vi "Dashboard Main.vi"() -> ()   [LabVIEW 2012]
uses:
  <vilib>/event_ctls.llb/eventvkey.ctl
  <vilib>/Utility/config.llb/Read Key (String).vi
  <vilib>/Utility/config.llb/Read Key (I32).vi
  <vilib>/Utility/config.llb/Write Key (String).vi
  <vilib>/Utility/config.llb/Write Key (I32).vi
  <vilib>/Utility/config.llb/NI_LVConfig.lvlib
panel:
  out "Mode":T1(ring)=enum."Auto Disabled"
  in  "Viewer":enum32{"Camera Image", "Variables"}(tab)
  out "Mbps":dbl format="%#.1g"
  in  "Enable":bool
  in  "DB Camera Config":bool
  out "Mbps":bool
  out "fps":dbl format="%#.1g"
  out "Image Error Message":string="Timeout in Camera Communications"
  out "Camera Image":T2(plugin-control)
  out "Camera Image 2":T2(plugin-control)
  in  "Camera Settings":T3={"Frame Rate"=15, "Compression"=30, "Size"=1} {"Frame Rate" scale=1.0..30.0; "Size" items=["640x480", "320x240", "160x120"]}
  out "Camera IP 2":string
  out "Camera IP":string
  out "fps 2":dbl format="%#.1g"
  out "Mbps 2":dbl format="%#.1g"
  in  "Enable 2":bool
  in  "FR":i32=15
  out "Tree":string(tree)
  in  "Dashboard Tab":enum32{"Operation", "Test", "Checklist"}(tab)
  in  "Slider":dbl(slide) scale=0.0..100.0 scale format="%#_3g"
  in  "On/Off":bool caption="Solenoid"
  in  "Test Name":u16(ring) items=["Select the test to run...", "Example Test", "-------------------------------", "List of tests is built in robot code.", "Replace with your own automated tests."]
  in  "Test Tree":string(tree)
  in  "Motor":cluster{"Value":dbl, "Enable":bool} {"Value" scale=-1.0..1.0 scale format="%#_3g"}
  out "Progress":T4 {"Test Progress" scale=0.0..100.0}
  in  "Rev/Fwd":cluster{"Forward":bool, "Reverse":bool}
  in  "Ring":u16(ring) items=["Auto", "Fixed indoor", "Fixed outdoor 1", "Fixed outdoor 2", "Fixed fluorescent 1", "Fixed fluorescent 2", "Hold current"]
  in  "Listbox":i32(listbox)
  out "Players":i8
  out "Skeleton Picture":picture
  out "Version":string
  out "Buttons 2":cluster{"1":bool, "2":bool, "3":bool}
  out "Kinect 2":cluster{"X":dbl, "Y":dbl, "Z":dbl} {"X" scale=1.0..-1.0; "Y" scale=1.0..-1.0; "Z" scale=1.0..-1.0}
  out "Buttons 1":cluster{"1":bool, "2":bool, "3":bool}
  out "Kinect 1":cluster{"X":dbl, "Y":dbl, "Z":dbl} {"X" scale=1.0..-1.0; "Y" scale=1.0..-1.0; "Z" scale=1.0..-1.0}
  out "Robot IP":string
  out "Battery Value":dbl(slide) scale=0.0..14.0 scale format="%#_2e"
  out "Battery":sgl(graph)
  # "Customize by placing controls and indicators here and name to match\nDashboard Variables on robot."
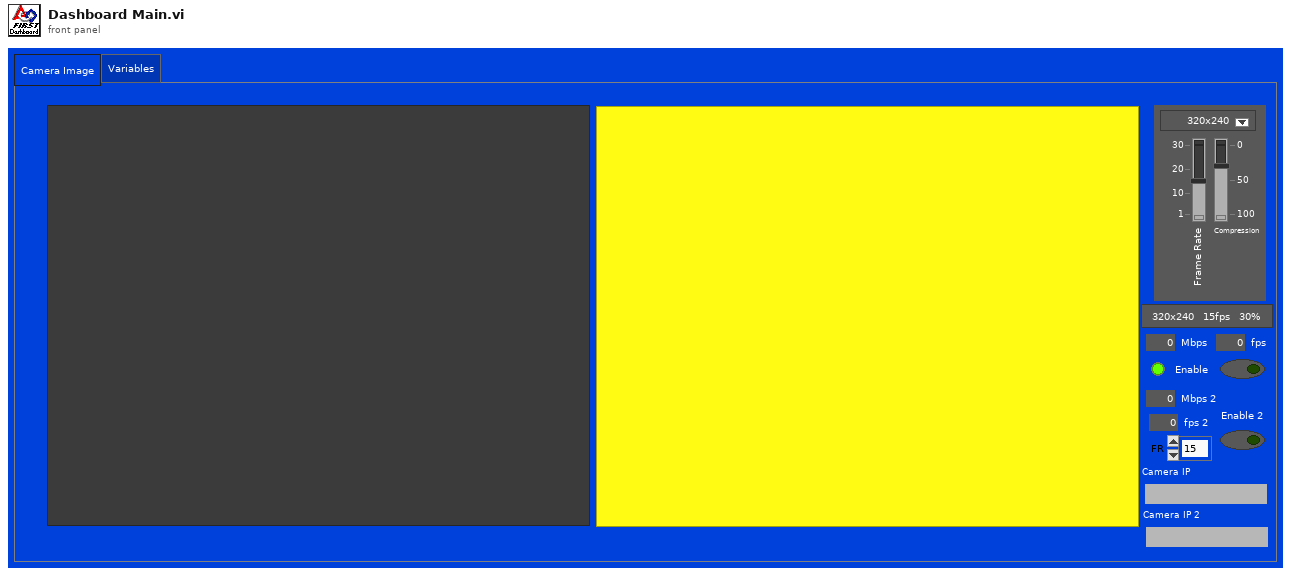
[diagram p1: front panel]
types:
  T1 = enum8{"Tele-Op Disabled", "Tele-Op Enabled", "Auto Disabled", "Auto Enabled", "Test Disabled", "Test Enabled", ""}
  T2 = typedef "IMAQ Image.ctl" = refnum<image>
  T3 = cluster{"Frame Rate":i32, "Compression":i32, "Size":u16}
  T4 = cluster{"Test Progress":u8, "Test Progress Text":string}
  T5 = typedef "Image Type" = u32
  T6 = typedef "LVBoundsTypeDef.ctl" = cluster{"Width":u32, "Height":u32}
  T7 = typedef "SkeletonTrackState.ctl" = enum32{"NotTracked", "PositionOnly", "Tracked"}
  T8 = cluster{"TrackingState":u8[], "Position":cluster{"x":sgl, "y":sgl, "z":sgl}, cluster{"x":sgl, "y":sgl, "z":sgl, sgl}[], "TrackState":T7}
  T9 = cluster{cluster{"ScaledToPercentRange":dbl, "ScaledToPercentRange":dbl, "ScaledToPercentRange":dbl}, cluster{bool, bool, bool}}[]
  T10 = cluster{cluster{"ScaledToPercentRange":dbl, "ScaledToPercentRange":dbl, "ScaledToPercentRange":dbl}, cluster{bool, bool, bool}}
  T11 = cluster{"ScaledToPercentRange":dbl, "ScaledToPercentRange":dbl, "ScaledToPercentRange":dbl}
  T12 = typedef "LVRectTypeDef.ctl" = cluster{"Left":i16, "Top":i16, "Right":i16, "Bottom":i16}
  T13 = cluster{"Competition mode":bool, "Robot Link":bool, "Autonomous":bool, "Enabled":bool, "E-Stop":bool, "Simulated":bool, "TestMode":bool, "Docked Window":bool}
  T14 = typedef "NI_LVConfig.lvlib/Config Data RefNum.ctl" = refnum<k1>
  T15 = typedef "eventvkey.ctl" = enum16{"ASCII", "Enter", "Return", "Shift", "Ctrl", "Alt", "Cmd", "Opt", "Caps", "NumLock", "Clear", "Break", "Up", "Down", "Left", "Right", "Insert", "Delete", "Home", "End", "PageUp", "PageDown", "Escape", "Help", "Pause", "ScrollLock", "F1", "F2", "F3", "F4", "F5", "F6", "F7", "F8", "F9", "F10", "F11", "F12", "F13", "F14", "F15", "F16", "F17", "F18", "F19", "F20", "F21", "F22", "F23", "F24", "Play", "VolumeUp", "VolumeDown", "Mute", "Two Byte Char"}
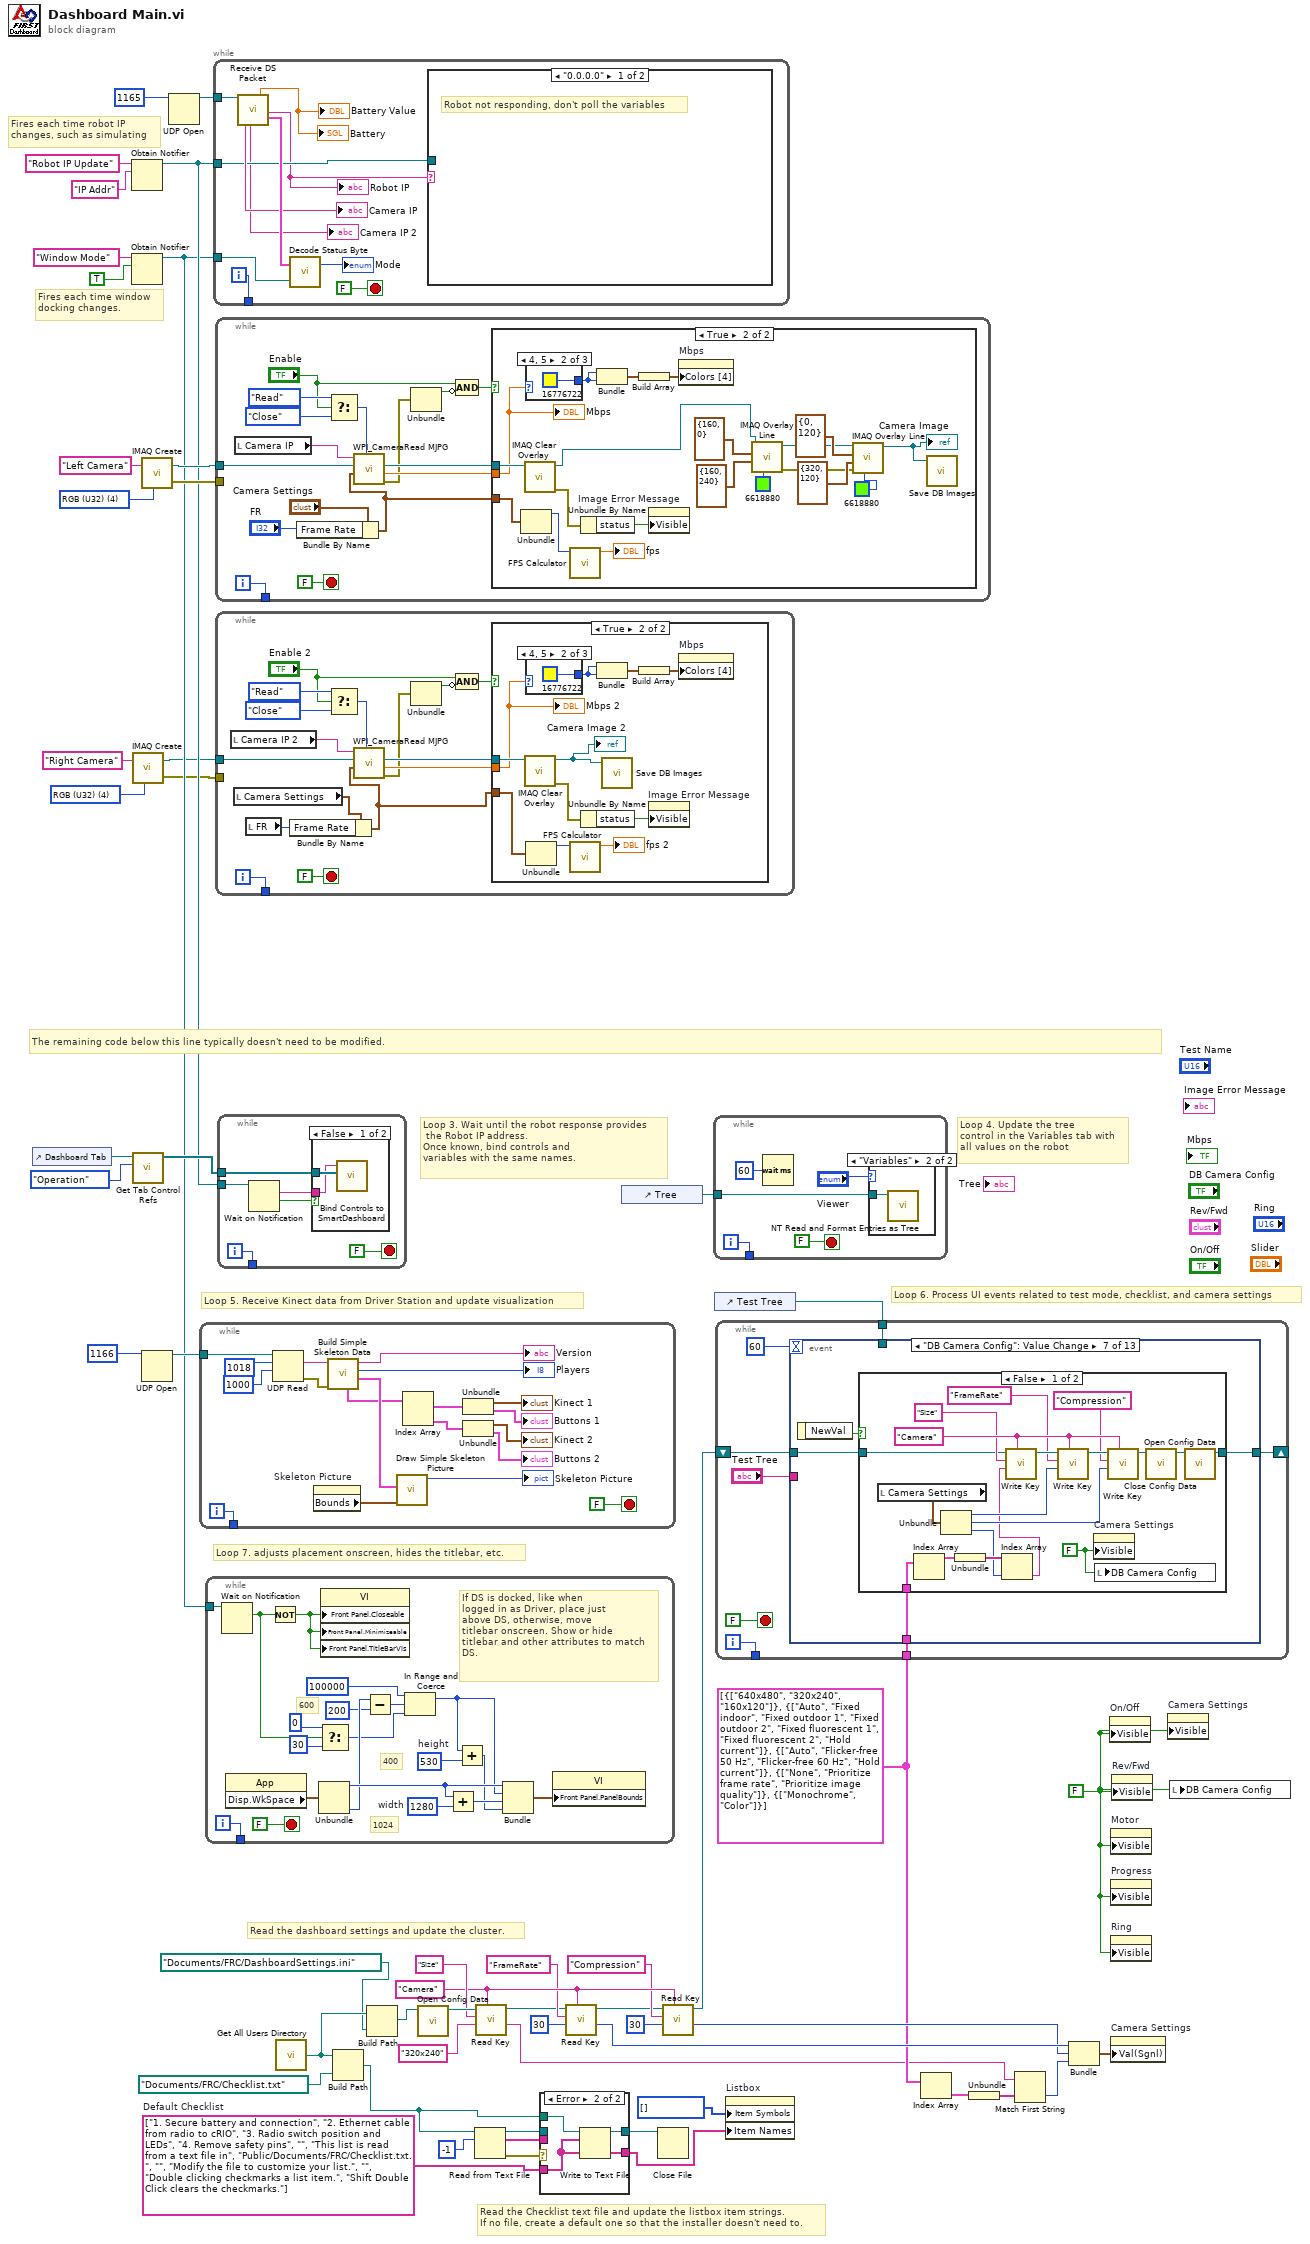
[diagram p0: block diagram]
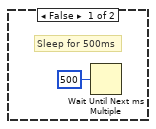
[diagram p2: hidden frame]
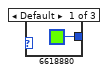
[diagram p3: hidden frame]
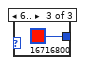
[diagram p4: hidden frame]
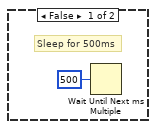
[diagram p6: hidden frame]
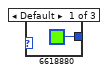
[diagram p7: hidden frame]
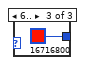
[diagram p8: hidden frame]
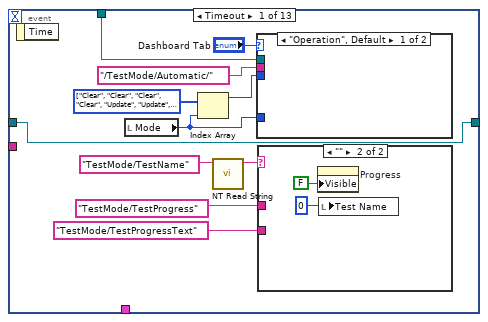
[diagram p10: hidden frame]
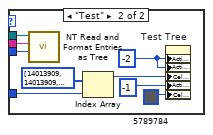
[diagram p11: hidden frame]
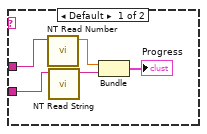
[diagram p12: hidden frame]
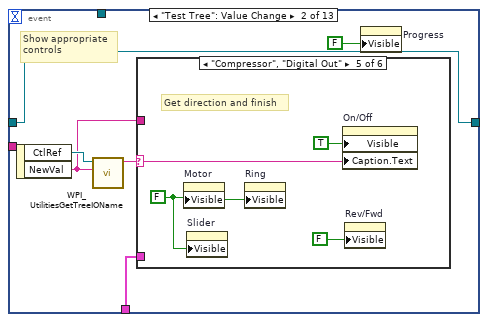
[diagram p13: hidden frame]
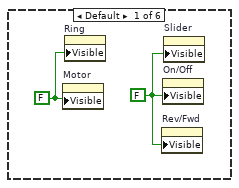
[diagram p14: hidden frame]
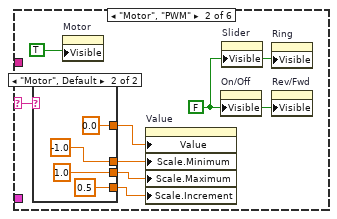
[diagram p15: hidden frame]
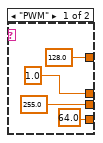
[diagram p16: hidden frame]
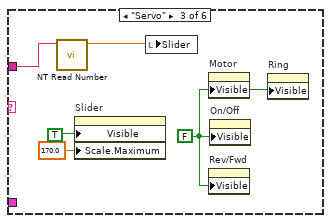
[diagram p17: hidden frame]
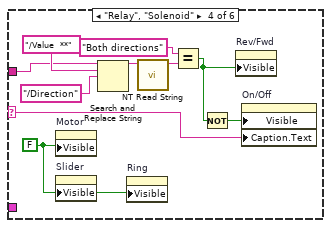
[diagram p18: hidden frame]
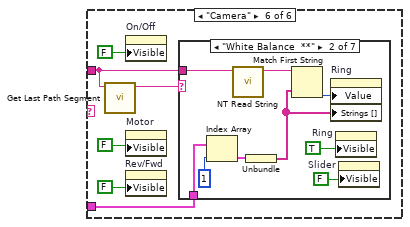
[diagram p19: hidden frame]
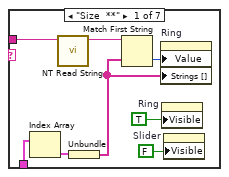
[diagram p20: hidden frame]
diagram:
  w3 = T5 4 items=["Grayscale (U8)", "Grayscale (I16)", "Grayscale (SGL)", "Complex (CSG)", "RGB (U32)", "HSL (U32)", "RGB (U64)"] ("Image Type")
  w25 = "Camera"
  w17 = cluster{string[]}[] [{["640x480", "320x240", "160x120"]}, {["Auto", "Fixed indoor", "Fixed outdoor 1", "Fixed outdoor 2", "Fixed fluorescent 1", "Fixed fluorescent 2", "Hold current"]}, {["Auto", "Flicker-free 50 Hz", "Flicker-free 60 Hz", "Hold current"]}, {["None", "Prioritize frame rate", "Prioritize image quality"]}, {["Monochrome", "Color"]}]
  w33 = string[] ["1. Secure battery and connection", "2. Ethernet cable from radio to cRIO", "3. Radio switch position and LEDs", "4. Remove safety pins", "", "This list is read from a text file in", "Public/Documents/FRC/Checklist.txt.", "", "Modify the file to customize your list.", "", "Double clicking checkmarks a list item.", "Shift Double Click clears the checkmarks."]  # Default Checklist
  w31 = FALSE ("Visible")
  w54 = T5 4 items=["Grayscale (U8)", "Grayscale (I16)", "Grayscale (SGL)", "Complex (CSG)", "RGB (U32)", "HSL (U32)", "RGB (U64)"] ("Image Type")
  # "Fires each time robot IP\nchanges, such as simulating"
  # "Fires each time window\ndocking changes."
  # "Read the Checklist text file and update the listbox item strings.\nIf no file, create a default one so that the installer doesn't need to."
  # "The remaining code below this line typically doesn't need to be modified."
  # "Loop 6. Process UI events related to test mode, checklist, and camera settings"
  # "Read the dashboard settings and update the cluster."
  # "Loop 4. Update the tree\ncontrol in the Variables tab with\nall values on the robot"
  # "Loop 3. Wait until the robot response provides\n the Robot IP address.\nOnce known, bind controls and\nvariables with the same names."
  # "Loop 5. Receive Kinect data from Driver Station and update visualization"
  # "Loop 7. adjusts placement onscreen, hides the titlebar, etc."
  n1 = control-ref of="Dashboard Tab"() -> (w47:refnum<vi>)
  n2 = Obtain Notifier(name (unnamed)="Robot IP Update", notification data type="IP Addr" ("name (unnamed)")) -> (notifier out=w44:refnum<notifier>)  [unwired: 2 in, 2 out]
  n3 = Obtain Notifier(name (unnamed)="Window Mode", notification data type=TRUE) -> (notifier out=w37:refnum<notifier>)  [unwired: 2 in, 2 out]
  n4 = call "IMAQ Create"("Image Name"="Right Camera", "Image Type"=w3) -> ("New Image"=w2:T2, "error out"=w1:errorcluster)  [unwired: 2 in, 1 out]
  n5 = call <vilib>:"Get Tab Control Refs.vi"("Page Index"=enum32{"Operation", "Test"}."Operation" ("Dashboard Tab"), "TabControl in"=w47) -> ("ControlsOnPage"=w48:refnum<vi>[])  [unwired: 9 in]
  n6 = call "IMAQ Create"("Image Name"="Left Camera", "Image Type"=w54) -> ("New Image"=w52:T2, "error out"=w51:errorcluster)  [unwired: 2 in, 1 out]
  n7 = UDP Open(11:u16 1166 ("port")) -> (port=w49:refnum<k16>)  [unwired: 2 in, 4 out]
  n8 = UDP Open(11:u16 1165 ("port")) -> (port=w55:refnum<k16>)  [unwired: 2 in, 4 out]
  n9 = while {
    tunnel: w49 -> [w73]
    tunnel: [w58] -> _
    i -> [w58]
    stop <- FALSE stop-if-true
    n10 = UDP Read(connection ID=w73, max size (548)=1018 ("bytes to read"), timeout ms (25000)=1000) -> (data out=w67:string, error out=w57:errorcluster)  [unwired: 1 in, 3 out]
    n11 = property on="Skeleton Picture" class="Pict"() -> ("Bounds"=w69:T6)  [unwired: 2 in, 2 out]
    n12 = call "Build Simple Skeleton Data.vi"("error in (no error)"=w57, "data in"=w67) -> ("Skeleton Data"=w68:T8, "NumPlayers"=→"Players":i8, "Version String"=→"Version":string, "Simple Joystick Info"=w65:T9)  [unwired: 5 in, 1 out]
    n13 = call "Draw Simple Skeleton Picture.vi"("Bounds"=w69, "Simple Skeleton"=w68) -> ("new picture out"=→"Skeleton Picture":picture)  [unwired: 9 in]
    n14 = Index Array(array=w65) -> (element #1=w64:T10, element #2=w63:T10)  [unwired: 2 in]
    n15 = Unbundle(w64) -> (→"Kinect 1":T11, →"Buttons 1":cluster{bool, bool, bool})
    n16 = Unbundle(w63) -> (→"Kinect 2":T11, →"Buttons 2":cluster{bool, bool, bool})
  }
  n17 = while {
    tunnel: w37 -> [w94]
    tunnel: [w92] -> _
    i -> [w92]
    stop <- FALSE stop-if-true
    w84 = 1280  # width
    w87 = 530  # height
    # "600"
    # "1024"
    # "400"
    # "If DS is docked, like when\nlogged in as Driver, place just\nabove DS, otherwise, move\ntitlebar onscreen. Show or hide\ntitlebar and other attributes to match\nDS."
    n18 = Wait on Notification(notifier=w94) -> (notification=w79:bool)  [unwired: 3 in, 3 out]
    n19 = property class="App"() -> ("Disp.WkSpace"=w90:T12)  [unwired: 2 in, 2 out]
    n20 = Not(x=w79) -> (.not. x?=w93:bool)
    n21 = Unbundle(w90) -> ("Left"=w88:i16, "Bottom"=w85:i16)  [unwired: 2 out]
    n22 = Select(t=0, s=w79, f=30) -> (s? t:f=w78:i32)
    n23 = property class="VI"("Front Panel.Closeable"=w93, "Front Panel.Minimizeable"=w93, "Front Panel.TitleBarVis"=w93) -> ()  [unwired: 2 in, 2 out]
    n24 = Subtract(x=w85, y=200) -> (x-y=w82:i32)
    n25 = In Range and Coerce(upper limit=100000, x=w82, lower limit=w78) -> (coerced(x)=w76:i32)  [unwired: 1 out]
    n26 = Add(x=w88, y=w84) -> (x+y=w89:i32)
    n27 = Add(x=w76, y=w87) -> (x+y=w86:i32)
    n28 = Bundle("Left"=w88, w76, w89, w86) -> (w91:cluster{"Left":i16, i32, i32, i32})  [unwired: 1 out]
    n29 = property class="VI"("Front Panel.PanelBounds"=w91) -> ()  [unwired: 2 in, 2 out]
  }
  n30 = while {
    tunnel: w55 -> [w104]
    tunnel: w44 -> [w98]
    tunnel: w37 -> [w102]
    tunnel: [w99] -> _
    i -> [w99]
    stop <- FALSE stop-if-true
    n31 = call "Receive DS Packet.vi"("Recv Socket"=w104) -> ("Camera IP Address"=→"Camera IP":string, "Camera IP Address 2"=→"Camera IP 2":string, "Battery"=→"Battery" →"Battery Value":sgl, "Robot IP Address"=w97:string, "Status"=w105:T13)  [unwired: 8 in, 6 out]
    "Robot IP" <- w97
    n32 = call "Decode Status Byte.vi"("Window Mode Notifier"=w102, "Status"=w105) -> ("Mode"=→"Mode":T1)  [unwired: 1 out]
    n33 = case shown="\"0.0.0.0\"" w97 {
      selector: w97 -> [_ w107]
      tunnel: w98 -> [_ w108]
      frame "0.0.0.0" {
        # "Robot not responding, don't poll the variables"
      }
      frame Default {
        # "Get info from Code"
        n34 = Send Notification(notification=w107, notifier=w108) -> ()  [unwired: 1 in, 2 out]
      }
    }
  }
  n35 = while {
    tunnel: w52 -> [w121]
    tunnel: w51 -> [_]
    tunnel: [w123] -> _
    i -> [w123]
    stop <- FALSE stop-if-true
    n36 = local read "Camera IP"() -> (w122:string)
    n37 = Bundle By Name(cluster="Camera Settings", "Frame Rate"="FR") -> (w109:T3)
    n38 = Select(t=enum16{"Read", "Reopen", "Close"}."Read" ("Operation"), s="Enable", f=enum16{"Read", "Reopen", "Close"}."Close" ("Operation")) -> (s? t:f=w116:enum16{"Read", "Reopen", "Close"})
    n39 = call <vilib>:"WPI_CameraRead MJPG.vi"("Operation"=w116, "Camera Settings"=w109, "Image"=w121, "address"=w122) -> ("error out"=w115:errorcluster, "Bandwidth (kbps)"=w119:dbl, "Image Out"=w120:T2)  [unwired: 5 in]
    n40 = Unbundle(w115) -> ("status"=w113:bool)  [unwired: 2 out]
    n41 = Compound Arithmetic op=AND("Enable", invert w113) -> (w112:bool)
    n42 = case shown="True" w112 {
      tunnel: w109 -> [_ w137]
      tunnel: w120 -> [_ w140]
      tunnel: w119 -> [_ w139]
      frame False {
        # "Sleep for 500ms"
        n43 = Wait Until Next ms Multiple(millisecond multiple=u32 500) -> ()  [unwired: 1 out]
      }
      frame True {
        n44 = Unbundle(w137) -> ("Frame Rate"=w127:i32)  [unwired: 2 out]
        n45 = call "IMAQ Clear Overlay"("Image"=w140) -> ("error out"=w144:errorcluster, "Image Out"=w129:T2)  [unwired: 2 in, 7 out]
        n46 = case shown="4, 5" w139 {
          tunnel: [u32 6618880 ("Color Box") u32 16776722 ("Color Box") u32 16716800 ("Color Box")] -> w141
          frame Default {
          }
          frame 4, 5 {
          }
          frame 6.. {
          }
        }
        n47 = call "FPS Calculator.vi"("Average Count"=w127) -> ("fps"=→"fps":dbl)  [unwired: 10 in]
        n48 = Unbundle By Name(w144) -> ("status"=w145:bool)
        n49 = Bundle("Color Box"=w141, "Color Box"=w141) -> (w143:cluster{"Color Box":u32, "Color Box":u32})  [unwired: 1 out]
        n50 = Build Array(w143) -> (w142:cluster{"Color Box":u32, "Color Box":u32}[])
        n51 = property on="Image Error Message" class="Str"("Visible"=w145) -> ()  [unwired: 2 in, 2 out]
        n52 = property on="Mbps" class="Bool (strict)"("Colors [4]"=w142) -> ()  [unwired: 2 in, 2 out]
        n53 = call "IMAQ Overlay Line"("Color"=u32 6618880, "End Point"=cluster{"X":i32, "Y":i32} {"X"=160, "Y"=240}, "Start Point"=cluster{"X":i32, "Y":i32} {"X"=160, "Y"=0}, "Image"=w129) -> ("error out"=w134:errorcluster, "Image Out"=w133:T2)  [unwired: 6 in]
        n54 = call "IMAQ Overlay Line"("Color"=u32 6618880, "error in (no error)"=w134, "End Point"=cluster{"X":i32, "Y":i32} {"X"=320, "Y"=120}, "Start Point"=cluster{"X":i32, "Y":i32} {"X"=0, "Y"=120}, "Image"=w133) -> ("Image Out"=w128:T2)  [unwired: 5 in, 1 out]
        "Camera Image" <- w128
        n55 = call "Save DB Images.vi"("Image"=w128) -> ()  [unwired: 2 in, 1 out]
        "Mbps" <- w139
      }
    }
  }
  n56 = while {
    tunnel: w2 -> [w161]
    tunnel: [w163] -> _
    tunnel: w1 -> [_]
    i -> [w163]
    stop <- FALSE stop-if-true
    n57 = local read "Camera IP 2"() -> (w162:string)
    n58 = local read "Camera Settings"() -> (w150:T3)
    n59 = local read "FR"() -> (w151:i32)
    n60 = Bundle By Name(cluster=w150, "Frame Rate"=w151) -> (w149:T3)
    n61 = Select(t=enum16{"Read", "Reopen", "Close"}."Read" ("Operation"), s="Enable 2", f=enum16{"Read", "Reopen", "Close"}."Close" ("Operation")) -> (s? t:f=w156:enum16{"Read", "Reopen", "Close"})
    n62 = call <vilib>:"WPI_CameraRead MJPG.vi"("Operation"=w156, "Camera Settings"=w149, "Image"=w161, "address"=w162) -> ("error out"=w155:errorcluster, "Bandwidth (kbps)"=w159:dbl, "Image Out"=w160:T2)  [unwired: 5 in]
    n63 = Unbundle(w155) -> ("status"=w153:bool)  [unwired: 2 out]
    n64 = Compound Arithmetic op=AND("Enable 2", invert w153) -> (w152:bool)
    n65 = case shown="True" w152 {
      tunnel: w149 -> [_ w168]
      tunnel: w160 -> [_ w171]
      tunnel: w159 -> [_ w170]
      frame False {
        # "Sleep for 500ms"
        n66 = Wait Until Next ms Multiple(millisecond multiple=u32 500) -> ()  [unwired: 1 out]
      }
      frame True {
        n67 = call "IMAQ Clear Overlay"("Image"=w171) -> ("error out"=w175:errorcluster, "Image Out"=w166:T2)  [unwired: 2 in, 7 out]
        "Camera Image 2" <- w166
        n68 = case shown="4, 5" w170 {
          tunnel: [u32 6618880 ("Color Box") u32 16776722 ("Color Box") u32 16716800 ("Color Box")] -> w172
          frame Default {
          }
          frame 4, 5 {
          }
          frame 6.. {
          }
        }
        n69 = Unbundle(w168) -> ("Frame Rate"=w167:i32)  [unwired: 2 out]
        n70 = call "FPS Calculator.vi"("Average Count"=w167) -> ("fps"=→"fps 2":dbl)  [unwired: 10 in]
        n71 = Unbundle By Name(w175) -> ("status"=w176:bool)
        n72 = Bundle("Color Box"=w172, "Color Box"=w172) -> (w174:cluster{"Color Box":u32, "Color Box":u32})  [unwired: 1 out]
        n73 = call "Save DB Images.vi"("Image"=w166) -> ()  [unwired: 2 in, 1 out]
        n74 = Build Array(w174) -> (w173:cluster{"Color Box":u32, "Color Box":u32}[])
        n75 = property on="Image Error Message" class="Str"("Visible"=w176) -> ()  [unwired: 2 in, 2 out]
        n76 = property on="Mbps" class="Bool (strict)"("Colors [4]"=w173) -> ()  [unwired: 2 in, 2 out]
        "Mbps 2" <- w170
      }
    }
  }
  n77 = while {
    tunnel: w48 -> [w185]
    tunnel: w44 -> [w182]
    tunnel: [w180] -> _
    i -> [w180]
    stop <- FALSE stop-if-true
    n78 = Wait on Notification(notifier=w182) -> (notification=w181:string, timed out?=w183:bool)  [unwired: 3 in, 2 out]
    n79 = case shown="False" w183 {
      tunnel: w185 -> [w187 _]
      tunnel: w181 -> [w186 _]
      frame False {
        n80 = call <vilib>:"Bind Controls to SmartDashboard.vi"("Bound Control Refs"=w187, "Server IP Address"=w186) -> ()  [unwired: 10 in]
      }
      frame True {
      }
    }
  }
  n81 = call "Get All Users Directory.vi"() -> ("All User Path"=w30:path)
  n82 = Build Path(base path=w30, name or relative path=path "Documents/FRC/Checklist.txt") -> (appended path=w34:path)
  n83 = Build Path(base path=w30, name or relative path=path "Documents/FRC/DashboardSettings.ini") -> (appended path=w29:path)
  n84 = call <vilib>:"Open Config Data.vi"("configuration file path"=w29) -> ("refnum"=w28:T14)  [unwired: 8 in, 2 out]
  n85 = Read from Text File(file (use dialog)=w34, count=-1 ("timeout ms (25000)")) -> (refnum out=w12:refnum<file>, text=w35:string[], error out=w36:errorcluster)  [unwired: 2 in, 1 out]
  n86 = call-poly <vilib>:"Read Key.vi"("section"=w25, "default value"="320x240", "key"="Size", "refnum"=w28) -> ("value"=w15:string, "refnum out"=w10:T14)  [unwired: 2 in, 4 out]
  n87 = case shown="Error" w36 {
    tunnel: w35 -> [w189 _]
    tunnel: [w189 w191] -> w32
    tunnel: w33 -> [_ w191]
    tunnel: w34 -> [_ w192]
    tunnel: [w188 w190] -> w11
    tunnel: w12 -> [w188 _]
    frame No Error {
    }
    frame Error {
      n88 = Write to Text File(file (use dialog)=w192, text=w191) -> (refnum out=w190:refnum<file>)  [unwired: 2 in, 2 out]
    }
  }
  n89 = call-poly <vilib>:"Read Key.vi"("section"=w25, "default value"=30, "key"="FrameRate", "refnum"=w10) -> ("value"=w20:i32, "refnum out"=w9:T14)  [unwired: 1 in, 5 out]
  n90 = control-ref of="Tree"() -> (w6:refnum<vi>)
  n91 = Close File(refnum=w11) -> ()  [unwired: 1 in, 2 out]
  n92 = call-poly <vilib>:"Read Key.vi"("section"=w25, "default value"=30, "key"="Compression", "refnum"=w9) -> ("value"=w19:i32, "refnum out"=w7:T14)  [unwired: 1 in, 5 out]
  n93 = while {
    tunnel: [w194] -> _
    tunnel: w6 -> [w193]
    i -> [w194]
    stop <- FALSE stop-if-true
    n94 = Wait (ms)(milliseconds to wait=u32 60) -> ()  [unwired: 1 out]
    n95 = case shown="\"Variables\"" "Viewer" {
      tunnel: w193 -> [_ w198]
      frame Default {
      }
      frame "Variables" {
        n96 = call <vilib>:"NT Read and Format Entries as Tree.vi"("Tree Refnum"=w198) -> ()  [unwired: 9 in, 2 out]
      }
    }
  }
  n97 = control-ref of="Test Tree"() -> (w5:refnum<vi>)
  n98 = while {
    tunnel: w17 -> [w203]
    shift-right: [w202] -> _
    shift-left: w7 -> [w201]
    tunnel: [w200] -> _
    tunnel: w5 -> [w199]
    i -> [w200]
    stop <- FALSE stop-if-true
    n99 = event shown="[6] \"DB Camera Config\": Value Change" {
      selector: _ -> [_ _ _ _ _ _ _ _ _ _ _ _ _]
      dyn-events: _ -> [_ _ _ _ _ _ _ _ _ _ _ _ _]
      timeout: u32 60 ("milliseconds to wait") -> [_ _ _ _ _ _ _ _ _ _ _ _ _]
      tunnel: w199 -> [w213 _ _ _ _ _ _ _ _ _ _ _ _]
      tunnel: "Test Tree" -> [_ _ _ _ _ _ _ _ w407 w415 w417 w421 w429]
      tunnel: w203 -> [_ w235 _ _ _ _ w371 w401 _ _ _ _ _]
      tunnel: [w207 w234 _ w337 w345 w357 w370 w394 w406 w413 w416 w420 w428] -> w202
      tunnel: w201 -> [w207 w234 _ w337 w345 w357 w369 w394 w406 w413 w416 w420 w428]
      event Timeout {
        w212 = enum16{"Update", "Clear"}[] [enum."Clear", enum."Clear", enum."Clear", enum."Clear", enum."Update", enum."Update", enum."Clear"] items=["Update", "Clear"]
        n100 = event-data() -> ()  [unwired: 1 in, 1 out]
        n101 = local read "Mode"() -> (w210:T1)
        n102 = Index Array(array=w212, index=w210) -> (element=w211:enum16{"Update", "Clear"})
        n103 = call <vilib>:"NT Read String.vi"("Name"="TestMode/TestName") -> ("String"=w216:string)  [unwired: 9 in, 1 out]
        n104 = case shown="\"Operation\", Default" "Dashboard Tab" {
          tunnel: w213 -> [_ w226]
          tunnel: "/TestMode/Automatic/" ("Name Pattern") -> [_ w225]
          tunnel: w211 -> [_ w224]
          tunnel: w210 -> [_ w222]
          frame "Operation", Default {
          }
          frame "Test" {
            w221 = -2 ("Active Item:Row Number")
            n105 = call <vilib>:"NT Read and Format Entries as Tree.vi"("Operation"=w224, "Name Pattern"=w225, "Tree Refnum"=w226) -> ()  [unwired: 7 in, 2 out]
            n106 = Index Array(array=u32[] [14013909, 14013909, 14013909, 14013909, 14013909, 16777215, 14013909], index=w222) -> (element=w220:u32)
            n107 = property on="Test Tree" class="Tree (strict)"("Active Item Row Number"=w221, "ActiveColNum"=w221, "CellBG"=w220, "Active Item Row Number"=-1 ("Active Item:Row Number"), "CellBG"=u32 5789784 ("Color Box")) -> ()  [unwired: 2 in, 2 out]
          }
        }
        n108 = case shown="\"\"" w216 {
          tunnel: "TestMode/TestProgress" ("Name") -> [w228 _]
          tunnel: "TestMode/TestProgressText" ("Name") -> [w227 _]
          frame Default {
            n109 = call <vilib>:"NT Read Number.vi"("Name"=w228) -> ("Numeric"=w229:dbl)  [unwired: 9 in, 1 out]
            n110 = call <vilib>:"NT Read String.vi"("Name"=w227) -> ("String"=w230:string)  [unwired: 9 in, 1 out]
            n111 = Bundle("Numeric"=w229, "String"=w230) -> (→"Progress":cluster{"Numeric":dbl, "String":string})  [unwired: 1 in]
          }
          frame "" {
            n112 = property on="Progress" class="Clust (strict)"("Visible"=FALSE) -> ()  [unwired: 2 in, 2 out]
            n113 = local write "Test Name"(u16 0) -> ()
          }
        }
      }
      event "Test Tree": Value Change {
        # "Show appropriate\ncontrols"
        n114 = event-data() -> ("CtlRef"=w238:refnum<vi>, "NewVal"=w236:string)  [unwired: 1 in]
        n115 = call <vilib>:"WPI_UtilitiesGetTreeIOName.vi"("NewVal"=w236, "TreeControl in"=w238) -> ("I/O Name"=w239:string)  [unwired: 9 in]
        n116 = case shown="\"Compressor\", \"Digital Out\"" w239 {
          selector: w239 -> [_ w246 _ w264 w273 _]
          tunnel: w236 -> [_ _ w261 w263 _ w280]
          tunnel: w235 -> [_ _ _ _ _ w279]
          frame Default {
            w241 = FALSE ("Visible")
            w240 = FALSE ("Visible")
            n117 = property on="Motor" class="Clust (strict)"("Visible"=w240) -> ()  [unwired: 2 in, 2 out]
            n118 = property on="Ring" class="Ring (strict)"("Visible"=w240) -> ()  [unwired: 2 in, 2 out]
            n119 = property on="Rev/Fwd" class="Clust (strict)"("Visible"=w241) -> ()  [unwired: 2 in, 2 out]
            n120 = property on="On/Off" class="Bool (strict)"("Visible"=w241) -> ()  [unwired: 2 in, 2 out]
            n121 = property on="Slider" class="Slide (strict)"("Visible"=w241) -> ()  [unwired: 2 in, 2 out]
          }
          frame "Motor", "PWM" {
            w247 = FALSE ("Visible")
            n122 = case shown="\"Motor\", Default" w246 {
              tunnel: [1.0 ("Value") -1.0 ("Value")] -> w245
              tunnel: [255.0 ("Value") 1.0 ("Value")] -> w244
              tunnel: [128.0 ("Value") 0.0 ("Value")] -> w243
              tunnel: [64.0 ("Value") 0.5 ("Value")] -> w242
              frame "PWM" {
              }
              frame "Motor", Default {
              }
            }
            n123 = property on="Motor" class="Clust (strict)"("Visible"=TRUE) -> ()  [unwired: 2 in, 2 out]
            n124 = property on="Value" class="Slide (strict)"("Value"=w243, "Scale.Minimum"=w245, "Scale.Maximum"=w244, "Scale.Increment"=w242) -> ()  [unwired: 2 in, 2 out]
            n125 = property on="On/Off" class="Bool (strict)"("Visible"=w247) -> ()  [unwired: 2 in, 2 out]
            n126 = property on="Slider" class="Slide (strict)"("Visible"=w247) -> ()  [unwired: 2 in, 2 out]
            n127 = property on="Ring" class="Ring (strict)"("Visible"=w247) -> ()  [unwired: 2 in, 2 out]
            n128 = property on="Rev/Fwd" class="Clust (strict)"("Visible"=w247) -> ()  [unwired: 2 in, 2 out]
          }
          frame "Servo" {
            w259 = FALSE ("Visible")
            n129 = call <vilib>:"NT Read Number.vi"("Name"=w261) -> ("Numeric"=w260:dbl)  [unwired: 9 in, 1 out]
            n130 = property on="Slider" class="Slide (strict)"("Visible"=TRUE, "Scale.Maximum"=170.0 ("Scale.Range:Maximum")) -> ()  [unwired: 2 in, 2 out]
            n131 = local write "Slider"(w260) -> ()
            n132 = property on="Motor" class="Clust (strict)"("Visible"=w259) -> ()  [unwired: 2 in, 2 out]
            n133 = property on="Rev/Fwd" class="Clust (strict)"("Visible"=w259) -> ()  [unwired: 2 in, 2 out]
            n134 = property on="On/Off" class="Bool (strict)"("Visible"=w259) -> ()  [unwired: 2 in, 2 out]
            n135 = property on="Ring" class="Ring (strict)"("Visible"=w259) -> ()  [unwired: 2 in, 2 out]
          }
          frame "Relay", "Solenoid" {
            w262 = FALSE ("Visible")
            n136 = property on="Motor" class="Clust (strict)"("Visible"=w262) -> ()  [unwired: 2 in, 2 out]
            n137 = property on="Slider" class="Slide (strict)"("Visible"=w262) -> ()  [unwired: 2 in, 2 out]
            n138 = Search and Replace String(input string=w263, search string="/Value  **", replace string="/Direction") -> (result string=w269:string)  [unwired: 5 in, 3 out]
            n139 = property on="Ring" class="Ring (strict)"("Visible"=w262) -> ()  [unwired: 2 in, 2 out]
            n140 = call <vilib>:"NT Read String.vi"("Name"=w269) -> ("String"=w267:string)  [unwired: 9 in, 1 out]
            n141 = Equal?(x="Both directions", y=w267) -> (x = y?=w265:bool)
            n142 = Not(x=w265) -> (.not. x?=w266:bool)
            n143 = property on="Rev/Fwd" class="Clust (strict)"("Visible"=w265) -> ()  [unwired: 2 in, 2 out]
            n144 = property on="On/Off" class="Bool (strict)"("Visible"=w266, "Caption.Text"=w264) -> ()  [unwired: 2 in, 2 out]
          }
          frame "Compressor", "Digital Out" {
            w272 = FALSE ("Visible")
            # "Get direction and finish"
            n145 = property on="Motor" class="Clust (strict)"("Visible"=w272) -> ()  [unwired: 2 in, 2 out]
            n146 = property on="Slider" class="Slide (strict)"("Visible"=w272) -> ()  [unwired: 2 in, 2 out]
            n147 = property on="Ring" class="Ring (strict)"("Visible"=w272) -> ()  [unwired: 2 in, 2 out]
            n148 = property on="On/Off" class="Bool (strict)"("Visible"=TRUE, "Caption.Text"=w273) -> ()  [unwired: 2 in, 2 out]
            n149 = property on="Rev/Fwd" class="Clust (strict)"("Visible"=FALSE) -> ()  [unwired: 2 in, 2 out]
          }
          frame "Camera" {
            n150 = call <vilib>:"Get Last Path Segment.vi"("String in"=w280) -> ("String out"=w281:string)  [unwired: 10 in]
            n151 = property on="On/Off" class="Bool (strict)"("Visible"=FALSE) -> ()  [unwired: 2 in, 2 out]
            n152 = property on="Motor" class="Clust (strict)"("Visible"=FALSE) -> ()  [unwired: 2 in, 2 out]
            n153 = property on="Rev/Fwd" class="Clust (strict)"("Visible"=FALSE) -> ()  [unwired: 2 in, 2 out]
            n154 = case shown="\"White Balance  **\"" w281 {
              tunnel: w280 -> [w287 w296 w305 w314 w323 _ w329]
              tunnel: w279 -> [w285 w293 w302 w311 w320 _ _]
              frame "Size  **" {
                n155 = Index Array(array=w285) -> (element=w284:cluster{string[]})  [unwired: 1 in]
                n156 = call <vilib>:"NT Read String.vi"("Name"=w287) -> ("String"=w286:string)  [unwired: 9 in, 1 out]
                n157 = Unbundle(w284) -> (w282:string[])
                n158 = Match First String(2:w282, 3:w286) -> (0:w283:i32)  [unwired: 1 out]
                n159 = property on="Ring" class="Ring (strict)"("Value"=w283, "Strings []"=w282) -> ()  [unwired: 2 in, 2 out]
                n160 = property on="Ring" class="Ring (strict)"("Visible"=TRUE) -> ()  [unwired: 2 in, 2 out]
                n161 = property on="Slider" class="Slide (strict)"("Visible"=FALSE) -> ()  [unwired: 2 in, 2 out]
              }
              frame "White Balance  **" {
                n162 = Index Array(array=w293, index=1) -> (element=w294:cluster{string[]})
                n163 = call <vilib>:"NT Read String.vi"("Name"=w296) -> ("String"=w295:string)  [unwired: 9 in, 1 out]
                n164 = Unbundle(w294) -> (w291:string[])
                n165 = Match First String(2:w291, 3:w295) -> (0:w290:i32)  [unwired: 1 out]
                n166 = property on="Ring" class="Ring (strict)"("Value"=w290, "Strings []"=w291) -> ()  [unwired: 2 in, 2 out]
                n167 = property on="Ring" class="Ring (strict)"("Visible"=TRUE) -> ()  [unwired: 2 in, 2 out]
                n168 = property on="Slider" class="Slide (strict)"("Visible"=FALSE) -> ()  [unwired: 2 in, 2 out]
              }
              frame "Exposure  **" {
                n169 = Index Array(array=w302, index=2) -> (element=w303:cluster{string[]})
                n170 = call <vilib>:"NT Read String.vi"("Name"=w305) -> ("String"=w304:string)  [unwired: 9 in, 1 out]
                n171 = Unbundle(w303) -> (w299:string[])
                n172 = Match First String(2:w299, 3:w304) -> (0:w300:i32)  [unwired: 1 out]
                n173 = property on="Ring" class="Ring (strict)"("Value"=w300, "Strings []"=w299) -> ()  [unwired: 2 in, 2 out]
                n174 = property on="Ring" class="Ring (strict)"("Visible"=TRUE) -> ()  [unwired: 2 in, 2 out]
                n175 = property on="Slider" class="Slide (strict)"("Visible"=FALSE) -> ()  [unwired: 2 in, 2 out]
              }
              frame "Exposure Priority  **" {
                n176 = Index Array(array=w311, index=3) -> (element=w312:cluster{string[]})
                n177 = call <vilib>:"NT Read String.vi"("Name"=w314) -> ("String"=w313:string)  [unwired: 9 in, 1 out]
                n178 = Unbundle(w312) -> (w308:string[])
                n179 = Match First String(2:w308, 3:w313) -> (0:w309:i32)  [unwired: 1 out]
                n180 = property on="Ring" class="Ring (strict)"("Value"=w309, "Strings []"=w308) -> ()  [unwired: 2 in, 2 out]
                n181 = property on="Ring" class="Ring (strict)"("Visible"=TRUE) -> ()  [unwired: 2 in, 2 out]
                n182 = property on="Slider" class="Slide (strict)"("Visible"=FALSE) -> ()  [unwired: 2 in, 2 out]
              }
              frame "Color Enable  **" {
                n183 = Index Array(array=w320, index=4) -> (element=w321:cluster{string[]})
                n184 = call <vilib>:"NT Read String.vi"("Name"=w323) -> ("String"=w322:string)  [unwired: 9 in, 1 out]
                n185 = Unbundle(w321) -> (w317:string[])
                n186 = Match First String(2:w317, 3:w322) -> (0:w318:i32)  [unwired: 1 out]
                n187 = property on="Ring" class="Ring (strict)"("Value"=w318, "Strings []"=w317) -> ()  [unwired: 2 in, 2 out]
                n188 = property on="Ring" class="Ring (strict)"("Visible"=TRUE) -> ()  [unwired: 2 in, 2 out]
                n189 = property on="Slider" class="Slide (strict)"("Visible"=FALSE) -> ()  [unwired: 2 in, 2 out]
              }
              frame Default {
                n190 = property on="Ring" class="Ring (strict)"("Visible"=FALSE) -> ()  [unwired: 2 in, 2 out]
                n191 = property on="Slider" class="Slide (strict)"("Visible"=FALSE) -> ()  [unwired: 2 in, 2 out]
              }
              frame "Brightness  **", "Color Level  **", "Compression  **", "FPS  **", "Sharpness  **" {
                n192 = call <vilib>:"NT Read Number.vi"("Name"=w329) -> ("Numeric"=w328:dbl)  [unwired: 9 in, 1 out]
                n193 = local write "Slider"(w328) -> ()
                n194 = property on="Slider" class="Slide (strict)"("Visible"=TRUE, "Scale.Maximum"=100.0 ("Scale.Range:Maximum")) -> ()  [unwired: 2 in, 2 out]
                n195 = property on="Ring" class="Ring (strict)"("Visible"=FALSE) -> ()  [unwired: 2 in, 2 out]
              }
            }
          }
        }
        n196 = property on="Progress" class="Clust (strict)"("Visible"=FALSE) -> ()  [unwired: 2 in, 2 out]
      }
      event "Test Name": Mouse Enter {
        # "Populate the ring with the list of tests"
        n197 = event-data() -> ()  [unwired: 1 in, 1 out]
        n198 = call <vilib>:"NT Read String Array.vi"("Name"="TestMode/TestList") -> ("String Array"=w336:string[])  [unwired: 9 in, 1 out]
        n199 = Build Array (concatenate)("Select the test to run...", w336) -> (w335:string[])
        n200 = property on="Test Name" class="Ring (strict)"("Strings []"=w335) -> ()  [unwired: 2 in, 2 out]
      }
      event "Test Name": Value Change {
        w338 = FALSE ("Visible")
        # "Tell the robot the test name to run"
        n201 = event-data() -> ("NewVal"=w342:u16)  [unwired: 1 in]
        n202 = property on="Test Name" class="Ring (strict)"() -> ("Strings []"=w343:string[])  [unwired: 2 in, 2 out]
        n203 = local write "Progress"(T4 {"Test Progress"=0, "Test Progress Text"=""} ("Progress")) -> ()
        n204 = Index Array(array=w343, index=w342) -> (element=w341:string)
        n205 = call <vilib>:"NT Write String.vi"("String"=w341, "Name"="TestMode/TestName") -> ()  [unwired: 9 in, 1 out]
        n206 = property on="Progress" class="Clust (strict)"("Visible"=TRUE) -> ()  [unwired: 2 in, 2 out]
        n207 = property on="Motor" class="Clust (strict)"("Visible"=w338) -> ()  [unwired: 2 in, 2 out]
        n208 = property on="Slider" class="Slide (strict)"("Visible"=w338) -> ()  [unwired: 2 in, 2 out]
        n209 = property on="On/Off" class="Bool (strict)"("Visible"=w338) -> ()  [unwired: 2 in, 2 out]
        n210 = property on="Rev/Fwd" class="Clust (strict)"("Visible"=w338) -> ()  [unwired: 2 in, 2 out]
        n211 = property on="Ring" class="Ring (strict)"("Visible"=w338) -> ()  [unwired: 2 in, 2 out]
      }
      event "Listbox": Double Click {
        n212 = event-data() -> ("PlatMods.Shift"=w346:bool, "Row"=w348:i32)  [unwired: 1 in]
        n213 = case shown="False" w346 {
          tunnel: w348 -> [w352 _]
          tunnel: 1 -> [w351 _]
          frame False {
            n214 = property on="Listbox" class="LstBox (strict)"() -> ("Item Symbols"=w350:i32[])  [unwired: 2 in, 2 out]
            n215 = Replace Array Subset(array=w350, new element=w351, index=w352) -> (w349:i32[])
            n216 = property on="Listbox" class="LstBox (strict)"("Item Symbols"=w349) -> ()  [unwired: 2 in, 2 out]
          }
          frame True {
            w353 = 0 ("Top Row")
            n217 = property on="Listbox" class="LstBox (strict)"() -> ("Number of Rows"=w355:u32)  [unwired: 2 in, 2 out]
            n218 = Initialize Array(0, w355) -> (w354:i32[])
            n219 = property on="Listbox" class="LstBox (strict)"("Top Row"=w353, "Value"=w353, "Item Symbols"=w354) -> ()  [unwired: 2 in, 2 out]
          }
        }
      }
      event "Listbox": Key Down {
        n220 = event-data() -> ("VKey"=w359:T15)  [unwired: 1 in]
        n221 = case shown="\"Left\", \"Right\"" w359 {
          selector: w359 -> [w364 _]
          tunnel: eventvkey."Left" ("VKey") -> [w362 _]
          frame "Left", "Right" {
            n222 = Equal?(x=w362, y=w364) -> (x = y?=w363:bool)
            n223 = Select(t=0, s=w363, f=1) -> (s? t:f=w365:i32)
            n224 = property on="Listbox" class="LstBox (strict)"() -> ("Item Symbols"=w368:i32[])  [unwired: 2 in, 2 out]
            n225 = Replace Array Subset(array=w368, new element=w365, index="Listbox") -> (w367:i32[])
            n226 = property on="Listbox" class="LstBox (strict)"("Item Symbols"=w367) -> ()  [unwired: 2 in, 2 out]
          }
          frame Default {
          }
        }
      }
      event "DB Camera Config": Value Change {
        n227 = event-data() -> ("NewVal"=w372:bool)  [unwired: 1 in]
        n228 = case shown="False" w372 {
          tunnel: w371 -> [w381 _]
          tunnel: [w374 w392] -> w370
          tunnel: w369 -> [w373 w392]
          frame False {
            w388 = "Camera"
            w391 = FALSE ("Visible")
            n229 = local read "Camera Settings"() -> (w380:T3)
            n230 = Index Array(array=w381) -> (element=w384:cluster{string[]})  [unwired: 1 in]
            n231 = Unbundle(w380) -> ("Frame Rate"=w379:i32, "Compression"=w378:i32, "Size"=w382:u16)
            n232 = Unbundle(w384) -> (w383:string[])
            n233 = Index Array(array=w383, index=w382) -> (element=w377:string)
            n234 = call-poly <vilib>:"Write Key.vi"("section"=w388, "value"=w377, "key"="Size", "refnum"=w373) -> ("refnum out"=w390:T14)  [unwired: 2 in, 5 out]
            n235 = call-poly <vilib>:"Write Key.vi"("section"=w388, "value"=w379, "key"="FrameRate", "refnum"=w390) -> ("refnum out"=w389:T14)  [unwired: 1 in, 6 out]
            n236 = property on="Camera Settings" class="Clust (strict)"("Visible"=w391) -> ()  [unwired: 2 in, 2 out]
            n237 = local write "DB Camera Config"(w391) -> ()
            n238 = call-poly <vilib>:"Write Key.vi"("section"=w388, "value"=w378, "key"="Compression", "refnum"=w389) -> ("refnum out"=w375:T14)  [unwired: 1 in, 6 out]
            n239 = call <vilib>:"Close Config Data.vi"("refnum"=w375) -> ("file path"=w376:path)  [unwired: 2 in, 8 out]
            n240 = call <vilib>:"Open Config Data.vi"("configuration file path"=w376) -> ("refnum"=w374:T14)  [unwired: 8 in, 2 out]
          }
          frame True {
            n241 = property on="Camera Settings" class="Clust (strict)"("Visible"=TRUE) -> ()  [unwired: 2 in, 2 out]
          }
        }
      }
      event "Camera Settings": Value Change {
        n242 = event-data() -> ("NewVal"=w405:T3)  [unwired: 1 in]
        n243 = Index Array(array=w401) -> (element=w400:cluster{string[]})  [unwired: 1 in]
        n244 = Unbundle(w405) -> ("Frame Rate"=w396:i32, "Compression"=w395:i32, "Size"=w398:u16)
        n245 = Unbundle(w400) -> (w399:string[])
        n246 = Index Array(array=w399, index=w398) -> (element=w397:string)
        n247 = Format Into String(format string="%s   %dfps   %d%%", w397, w396, w395) -> (resulting string=w402:string)  [unwired: 2 in, 1 out]
        n248 = Build Array(w402) -> (w403:string[])
        n249 = property on="DB Camera Config" class="Bool (strict)"("Strings [4]"=w403) -> ()  [unwired: 2 in, 2 out]
      }
      event "Motor.Enable": Value Change {
        n250 = event-data() -> ("NewVal"=w411:bool)  [unwired: 1 in]
        n251 = Unbundle("Motor") -> ("Value"=w410:dbl)  [unwired: 1 out]
        n252 = Select(t=w410, s=w411, f=0.0) -> (s? t:f=w408:dbl)
        n253 = call <vilib>:"NT Write Number.vi"("Numeric"=w408, "Name"=w407) -> ()  [unwired: 9 in, 1 out]
      }
      event "Slider": Value Change {
        n254 = event-data() -> ("NewVal"=w414:dbl)  [unwired: 1 in]
        n255 = call <vilib>:"NT Write Number.vi"("Numeric"=w414, "Name"=w415) -> ()  [unwired: 9 in, 1 out]
      }
      event "On/Off": Value Change {
        n256 = event-data() -> ("NewVal"=w419:bool)  [unwired: 1 in]
        n257 = Boolean To (0,1)(Boolean=w419) -> (0, 1=w418:i16)
        n258 = call <vilib>:"NT Write Number.vi"("Numeric"=w418, "Name"=w417) -> ()  [unwired: 9 in, 1 out]
      }
      event "Rev/Fwd": Value Change {
        n259 = event-data() -> ("NewVal.Forward"=w427:bool, "NewVal.Reverse"=w426:bool)  [unwired: 1 in]
        n260 = Boolean To (0,1)(Boolean=w427) -> (0, 1=w423:i16)
        n261 = Boolean To (0,1)(Boolean=w426) -> (0, 1=w425:i16)
        n262 = Negate(x=w425) -> (-x=w424:i16)
        n263 = Add(x=w423, y=w424) -> (x+y=w422:i16)
        n264 = call <vilib>:"NT Write Number.vi"("Numeric"=w422, "Name"=w421) -> ()  [unwired: 9 in, 1 out]
      }
      event "Ring": Value Change {
        n265 = event-data() -> ("NewVal"=w431:u16)  [unwired: 1 in]
        n266 = property on="Ring" class="Ring (strict)"() -> ("Strings []"=w432:string[])  [unwired: 2 in, 2 out]
        n267 = Index Array(array=w432, index=w431) -> (element=w430:string)
        n268 = call <vilib>:"NT Write String.vi"("String"=w430, "Name"=w429) -> ()  [unwired: 9 in, 1 out]
      }
    }
  }
  n269 = property on="Listbox" class="LstBox (strict)"("Item Symbols"=i32[] [], "Item Names"=w32) -> ()  [unwired: 2 in, 2 out]
  n270 = Index Array(array=w17) -> (element=w18:cluster{string[]})  [unwired: 1 in]
  n271 = Unbundle(w18) -> (w16:string[])
  n272 = Match First String(2:w16, 3:w15) -> (0:w14:i32)  [unwired: 1 out]
  n273 = Bundle("value"=w20, "value"=w19, "index"=w14) -> (w8:cluster{"value":i32, "value":i32, "index":i32})  [unwired: 1 out]
  n274 = property on="On/Off" class="Bool (strict)"("Visible"=w31) -> ()  [unwired: 2 in, 2 out]
  n275 = property on="Motor" class="Clust (strict)"("Visible"=w31) -> ()  [unwired: 2 in, 2 out]
  n276 = property on="Progress" class="Clust (strict)"("Visible"=w31) -> ()  [unwired: 2 in, 2 out]
  n277 = property on="Ring" class="Ring (strict)"("Visible"=w31) -> ()  [unwired: 2 in, 2 out]
  n278 = property on="Camera Settings" class="Clust (strict)"("Val(Sgnl)"=w8) -> ()  [unwired: 2 in, 2 out]
  n279 = property on="Rev/Fwd" class="Clust (strict)"("Visible"=w31) -> ()  [unwired: 2 in, 2 out]
  n280 = property on="Camera Settings" class="Clust (strict)"("Visible"=w31) -> ()  [unwired: 2 in, 2 out]
  n281 = local write "DB Camera Config"(w31) -> ()
